vi "Launcher.vi"   [LabVIEW 2021]
uses:
  User Event/UE Control.ctl
  User Event/User Event.lvlib
  Controller/EOL Controller.lvlib
  User Interface/User Console.lvlib
  Display Console/Display Console.lvlib
  Network/Network.lvlib
  IO Interface/IO Interface.lvlib
  Config Database/Config Database.lvlib
  Error Handling/Error Handling.lvlib
panel:
  # "This VI is the Launcher for EOL Test System \n\nThis VI performs any actions required to occur before the modules begin running or after they close \n(such as creating the user events). \nIt then launches the modules. The UI is launched dynamically when the program is run."
types:
  T1 = typedef "User Event.lvlib/UE Control.ctl" = enum16{"Create", "Get", "Generate", "Destroy"}
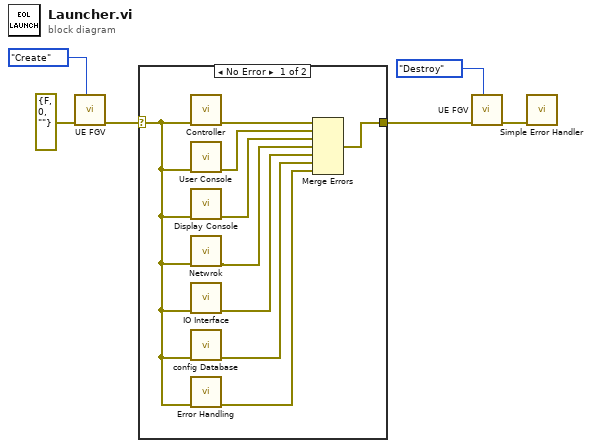
[diagram p0: block diagram]
diagram:
  n1 = call "UE FGV.vi"("UE Ctls"=UE_Control."Create", "error in (no error)"=errorcluster {"status"=FALSE, "code"=0, "source"=""}) -> ("error out"=w6:errorcluster)  [unwired: 8 in, 1 out]
  n2 = case shown="No Error" w6 {
    selector: w6 -> [w11 w16]
    tunnel: [w15 w16] -> w3
    frame No Error {
      n3 = call "Controller.vi"("error in (no error)"=w11) -> ("error out"=w14:errorcluster)  [unwired: 10 in]
      n4 = call "User Console.vi"("error in (no error)"=w11) -> ("error out"=w13:errorcluster)  [unwired: 10 in]
      n5 = call "Display Console.vi"("error in (no error)"=w11) -> ("error out"=w12:errorcluster)  [unwired: 10 in]
      n6 = call "Netwrok.vi"("error in (no error)"=w11) -> ("error out"=w10:errorcluster)  [unwired: 10 in]
      n7 = call "IO Interface.vi"("error in (no error)"=w11) -> ("error out"=w9:errorcluster)  [unwired: 10 in]
      n8 = call "config Database.vi"("error in (no error)"=w11) -> ("error out"=w8:errorcluster)  [unwired: 10 in]
      n9 = call "Error Handling.vi"("error in (no error)"=w11) -> ("error out"=w7:errorcluster)  [unwired: 10 in]
      n10 = Merge Errors(w14, w13, w12, w10, w9, w8, w7) -> (w15:errorcluster)
    }
    frame Error {
    }
  }
  n11 = call "UE FGV.vi"("UE Ctls"=UE_Control."Destroy", "error in (no error)"=w3) -> ("error out"=w1:errorcluster)  [unwired: 8 in, 1 out]
  n12 = call <vilib>:"Simple Error Handler.vi"("error in (no error)"=w1) -> ()  [unwired: 4 in, 5 out]
